vi "cut xy graph using x values.vi"(3 "x_max":sgl, 4 "x_min":sgl, 5 "f(x)":dbl[](array[numeric]), 6 "x":dbl[](array[numeric])) -> (0 "y_cut":dbl[](array[numeric]), 1 "x_cut":dbl[](array[numeric]), 2 "index of start of cut":i32)   [LabVIEW 2020]
panel:
  out "fractional index or x":dbl
  out "index of end cut":i32
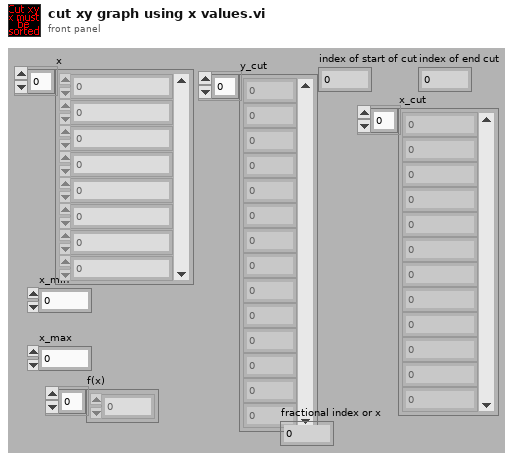
[diagram p1: front panel]
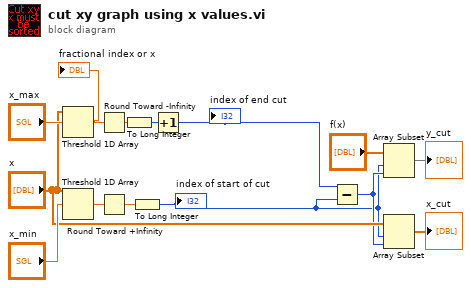
[diagram p0: block diagram]
diagram:
  n1 = Threshold 1D Array(2:"x_max", 3:"x") -> (0:w10:dbl)  [unwired: 1 out]
  "fractional index or x" <- w10
  n2 = Threshold 1D Array(2:"x_min", 3:"x") -> (0:w6:dbl)  [unwired: 1 out]
  n3 = Round Toward -Infinity(1:w10) -> (0:w4:dbl)
  n4 = Round Toward +Infinity(x=w6) -> (ceil(x): smallest int >= x=w5:dbl)
  n5 = To Long Integer(number=w4) -> (32bit integer=w3:i32)
  n6 = To Long Integer(number=w5) -> (32bit integer=w2:i32)
  "index of start of cut" <- w2
  n7 = Increment(x=w3) -> (x+1=w1:i32)
  "index of end cut" <- w1
  n8 = Subtract(x=w1, y=w2) -> (x-y=w11:i32)
  n9 = Array Subset(array="f(x)", index=w2, length=w11) -> (→"y_cut":dbl[])
  n10 = Array Subset(array="x", index=w2, length=w11) -> (→"x_cut":dbl[])
